vi "Read Config.vi"(8 "error in (no error)":errorcluster, 11 "AcquistionObject in":refnum<class "AcquistionObject.lvclass">) -> (0 "error out":errorcluster, 2 "config data":T1, 3 "AcquistionObject out":refnum<class "AcquistionObject.lvclass">)   [LabVIEW 2014, in "AcquisitionCoreObjects.lvlib" / "AcquistionObject.lvclass"]
uses:
  AcquistionObject.lvclass
  <vilib>/Utility/config.llb/Config Data RefNum.ctl
  AcquistionObject.lvclass/AcquistionObject.ctl
  <vilib>/Utility/config.llb/NI_LVConfig.lvlib
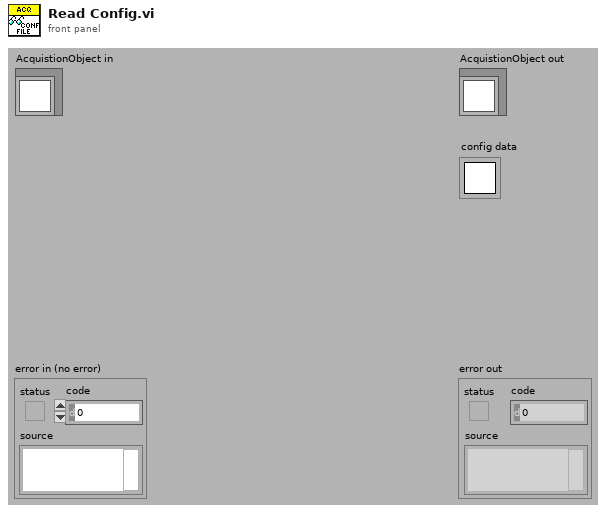
[diagram p1: front panel]
types:
  T1 = typedef "NI_LVConfig.lvlib/Config Data RefNum.ctl" = refnum<k1>
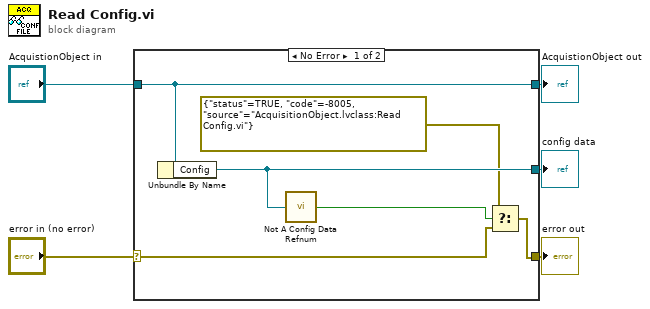
[diagram p0: block diagram]
diagram:
  n1 = case shown="No Error" "error in (no error)" {
    selector: "error in (no error)" -> [w7 w12]
    tunnel: [w6 w12] -> w4
    tunnel: [w11 w13] -> w2
    tunnel: "AcquistionObject in" -> [w11 w13]
    tunnel: [w10 _] -> w1
    frame No Error {
      n2 = Unbundle By Name(w11) -> ("Config"=w10:T1)
      n3 = call <vilib>:"Not A Config Data Refnum.vi"("refnum"=w10) -> ("not a config data refnum"=w9:bool)
      n4 = Select(t=errorcluster {"status"=TRUE, "code"=-8005, "source"="AcquisitionObject.lvclass:Read Config.vi"} ("f"), s=w9, f=w7) -> (s? t:f=w6:errorcluster)
    }
    frame Error {
    }
  }
  "error out" <- w4
  "AcquistionObject out" <- w2
  "config data" <- w1
